vi "WriteStageSettings.vi"(1 "error in (no error)":errorcluster) -> (0 "error out":errorcluster)   [LabVIEW 2009]
uses:
  Write Key (I32).vi
  <vilib>/Utility/config.llb/NI_LVConfig.lvlib
panel:
  in  "Case Constant\n(See Context Help)":bool
  in  "VI Refnum":refnum<vi>
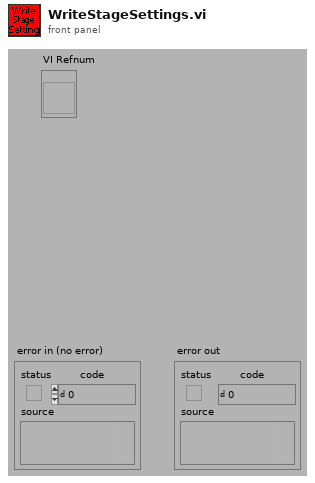
[diagram p1: front panel]
types:
  T1 = enum16{"Get Type", "Set Type", "GetStageInit", "GetWriteStageSetting", "GetInitializeStageOutput", "GetSetAxisPosition", "GetSetPos"}
  T2 = typedef "NI_LVConfig.lvlib/Config Data RefNum.ctl" = refnum<k1>
  T3 = typedef "StageType.ctt" = enum16{"PI analogue", "PI 712 TCP/IP", "Märzhäuser", "PI analogue step"}
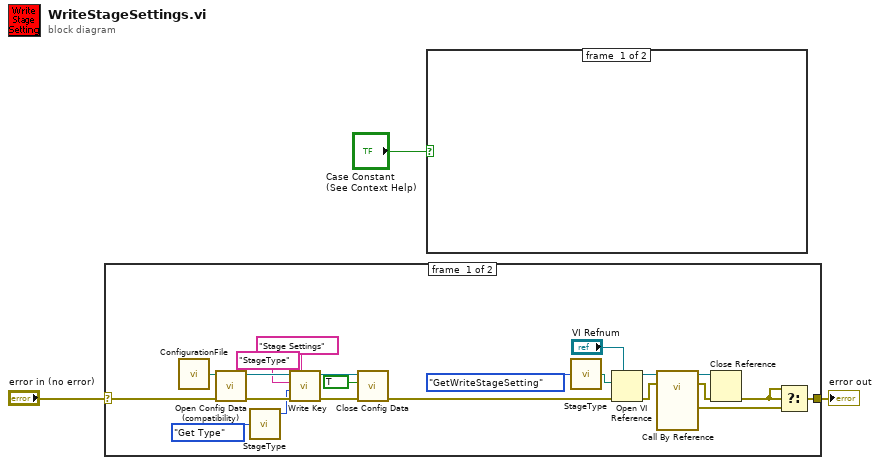
[diagram p0: block diagram]
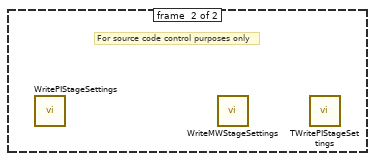
[diagram p2: hidden frame]
diagram:
  n1 = case shown="No Error" "error in (no error)" {
    selector: "error in (no error)" -> [w14 w26]
    tunnel: [w16 w26] -> w2
    frame #0 {
      n2 = call "ConfigurationFile.vi"() -> ("Configuration File (output)"=w15:path)  [unwired: 2 in]
      n3 = call <vilib>:"Open Config Data (compatibility).vi"("error in (no error)"=w14, "configuration file path"=w15) -> ("error out"=w12:errorcluster, "refnum"=w13:T2)  [unwired: 7 in, 1 out]
      n4 = call "StageType.vi"("Function"=T1."Get Type") -> ("Stage Type (output)"=w8:T3)  [unwired: 2 in, 2 out]
      n5 = call-poly "Write Key.vi"("section"="Stage Settings", "error in (no error)"=w12, "value"=w8, "key"="StageType", "refnum"=w13) -> ("error out"=w6:errorcluster, "refnum out"=w7:T2)  [unwired: 5 in]
      n6 = call "Close Config Data.vi"("error in (no error)"=w6, "write configuration file? (T)"=TRUE ("write configuration file? (F)"), "refnum"=w7) -> ("error out"=w4:errorcluster)  [unwired: 8 in]
      n7 = call "StageType.vi"("Function"=T1."GetWriteStageSetting") -> ("VI Path"=w24:path)  [unwired: 2 in, 2 out]
      n8 = Open VI Reference(type specifier VI Refnum (for type only)="VI Refnum", vi path=w24, error in (no error)=w4) -> (vi reference=w23:refnum<vi>, error out=w22:errorcluster)  [unwired: 3 in]
      n9 = call-by-ref "?"(reference=w23, error in=w22) -> (reference out=w21:refnum<vi>, error out=w20:errorcluster, 0:"error out"=w18:errorcluster)  [unwired: 1 in]
      n10 = Close Reference(reference=w21, error in (no error)=w20) -> (error out=w19:errorcluster)
      n11 = Select(t=w19, s=w19, f=w18) -> (s? t:f=w16:errorcluster)
    }
    frame #1 {
    }
  }
  "error out" <- w2
  n12 = case shown="True" "Case Constant\n(See Context Help)" {
    frame #0 {
    }
    frame #1 {
      # "For source code control purposes only"
      n13 = call "WritePIStageSettings.vi"() -> ()  [unwired: 1 in, 1 out]
      n14 = call "WriteMWStageSettings.vi"() -> ()  [unwired: 1 in, 1 out]
      n15 = call "TWritePIStageSettings.vi"() -> ()  [unwired: 1 in, 1 out]
    }
  }
